vi "decodeMapHeader.vi"(8 "error in (no error)":errorcluster, 11 "ByteArray":u8[](array[numeric]) format="%x") -> (0 "error out":errorcluster, 3 "RemainingBytes":u8[](array[numeric]) format="%x", 5 "Type":string, 7 "Map Size":u32)   [LabVIEW 2015, in "MsgPack.lvlib"]
uses:
  MsgPack.lvlib
  <vilib>/ErrorRing/Error Ring.xnode
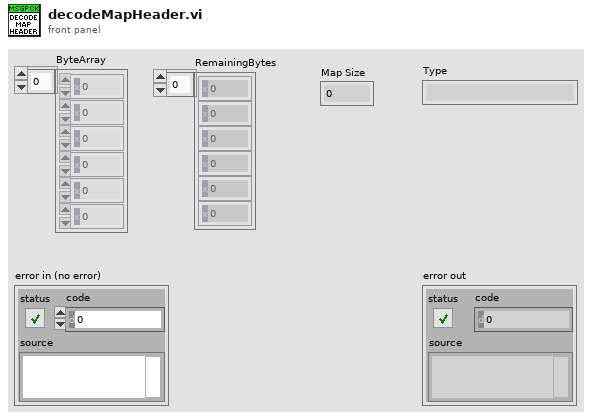
[diagram p1: front panel]
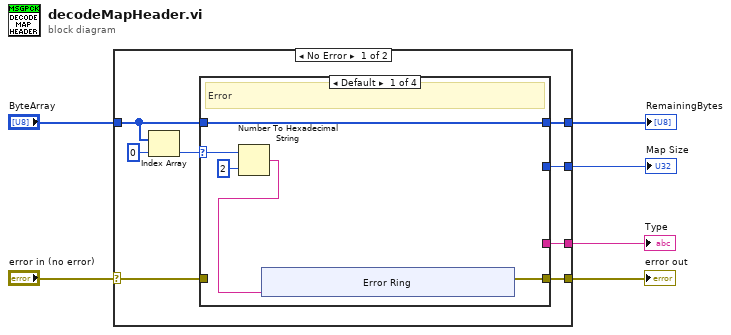
[diagram p0: block diagram]
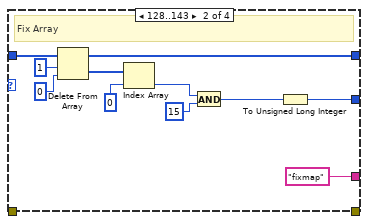
[diagram p2: hidden frame]
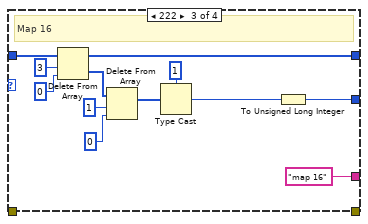
[diagram p3: hidden frame]
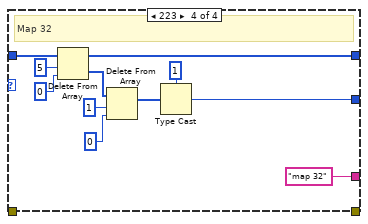
[diagram p4: hidden frame]
diagram:
  n1 = case shown="No Error" "error in (no error)" {
    selector: "error in (no error)" -> [w12 w60]
    tunnel: [w14 w60] -> w6
    tunnel: [w13 _] -> w5
    tunnel: "ByteArray" -> [w10 w59]
    tunnel: [w11 w59] -> w3
    tunnel: [w7 _] -> w1
    frame No Error {
      n2 = Index Array(array=w10, index=0) -> (element=w9:u8)
      n3 = case shown="Default" w9 {
        selector: w9 -> [w16 _ _ _]
        tunnel: [w18 _ _ _] -> w14
        tunnel: w12 -> [_ _ _ _]
        tunnel: [_ "fixmap" "map 16" "map 32"] -> w13
        tunnel: [w19 w29 w38 w48] -> w11
        tunnel: w10 -> [w19 w33 w45 w56]
        tunnel: [_ w25 w36 w49] -> w7
        frame Default {
          # "Error"
          n4 = Number To Hexadecimal String(1:i16 2 ("width (-)"), 2:w16) -> (0:w15:string)
          n5 = xnode "Error Ring"("parameter 0"=w15) -> ("error out"=w18:errorcluster)
        }
        frame 128..143 {
          # "Fix Array"
          n6 = Delete From Array(array=w33, length=1, index=0) -> (deleted portion=w31:u8[], array with subset deleted=w29:u8[])
          n7 = Index Array(array=w31, index=0) -> (element=w27:u8)
          n8 = And(x=w27, y=u8 15) -> (x .and. y?=w26:u8)
          n9 = To Unsigned Long Integer(number=w26) -> (unsigned 32bit integer=w25:u32)
        }
        frame 222 {
          # "Map 16"
          n10 = Delete From Array(array=w45, length=3, index=0) -> (deleted portion=w42:u8[], array with subset deleted=w38:u8[])
          n11 = Delete From Array(array=w42, length=1, index=0) -> (array with subset deleted=w41:u8[])  [unwired: 1 out]
          n12 = Type Cast(type=u16 1 ("index"), x=w41) -> (*(type *) &x=w37:u16)
          n13 = To Unsigned Long Integer(number=w37) -> (unsigned 32bit integer=w36:u32)
        }
        frame 223 {
          # "Map 32"
          n14 = Delete From Array(array=w56, length=5, index=0) -> (deleted portion=w53:u8[], array with subset deleted=w48:u8[])
          n15 = Delete From Array(array=w53, length=1, index=0) -> (array with subset deleted=w52:u8[])  [unwired: 1 out]
          n16 = Type Cast(type=u32 1 ("index"), x=w52) -> (*(type *) &x=w49:u32)
        }
      }
    }
    frame Error {
    }
  }
  "error out" <- w6
  "Type" <- w5
  "RemainingBytes" <- w3
  "Map Size" <- w1
